vi "Handle Remote Command.vi"(8 "error in (no error)":errorcluster, 9 "Data":string, 10 "Command":string, 11 "Instrument in":refnum<class "Instrument.lvclass">) -> (0 "error out":errorcluster, 2 "String":string, 3 "Instrument out":refnum<class "Instrument.lvclass">)   [LabVIEW 2016, in "Instrument.lvclass"]
uses:
  Instrument.lvclass
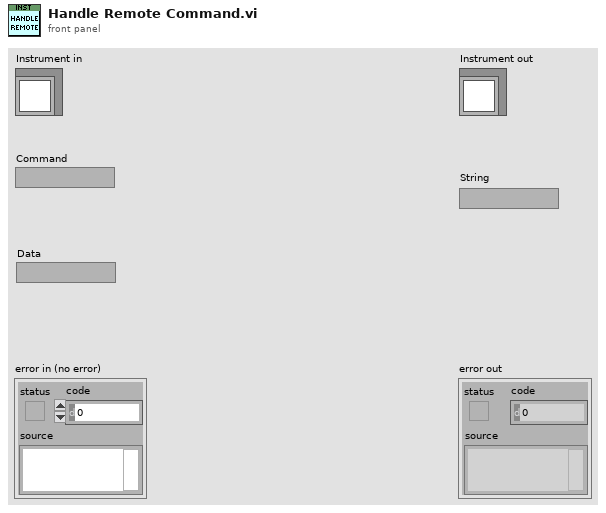
[diagram p1: front panel]
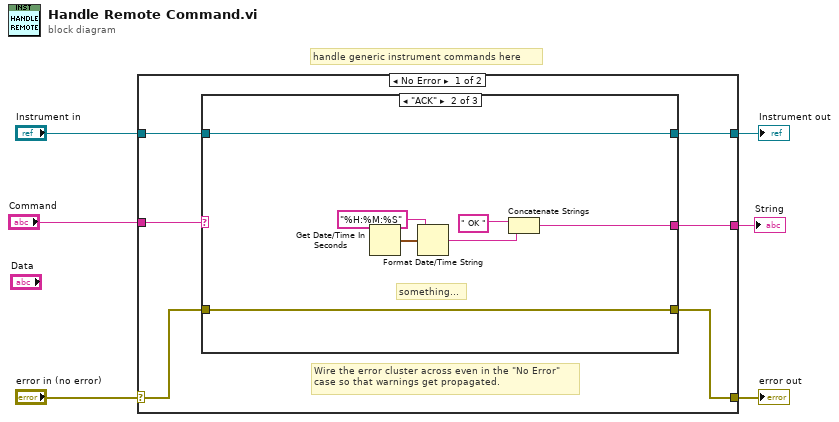
[diagram p0: block diagram]
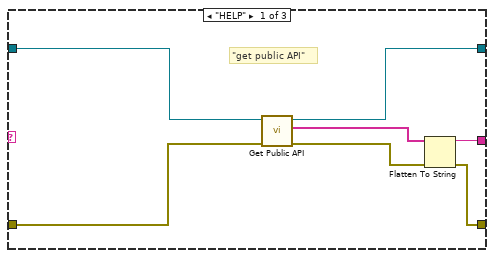
[diagram p2: hidden frame]
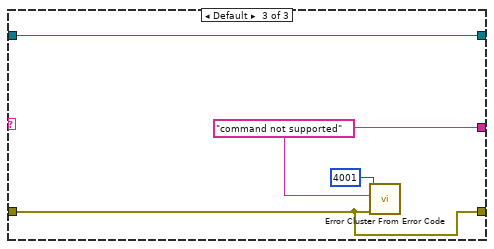
[diagram p3: hidden frame]
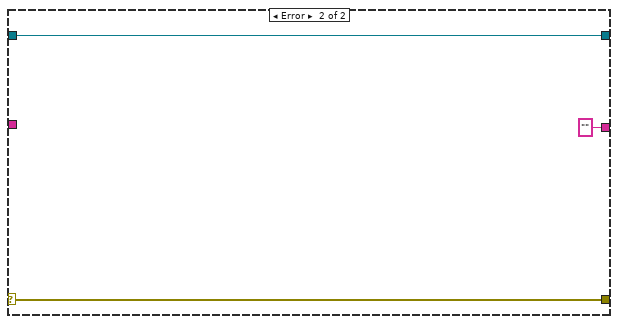
[diagram p4: hidden frame]
diagram:
  # "handle generic instrument commands here"
  n1 = case shown="No Error" "error in (no error)" {
    selector: "error in (no error)" -> [w8 w33]
    tunnel: [w7 w33] -> w5
    tunnel: [w10 w32] -> w3
    tunnel: "Instrument in" -> [w11 w32]
    tunnel: "Command" -> [w12 _]
    tunnel: [w9 "" ("error message (\"\")")] -> w1
    frame No Error {
      # "Wire the error cluster across even in the \"No Error\"\ncase so that warnings get propagated."
      n2 = case shown="\"ACK\"" w12 {
        tunnel: w11 -> [w19 w26 w29]
        tunnel: [w18 w26 w29] -> w10
        tunnel: [w15 w20 w27] -> w9
        tunnel: w8 -> [w17 w21 w28]
        tunnel: [w13 w21 w28] -> w7
        frame "HELP" {
          # "\"get public API\""
          n3 = call-dynamic "Get Public API.vi"("error in (no error)"=w17, "Instrument in"=w19) -> ("error out"=w14:errorcluster, "Commands"=w16:string[], "Instrument out"=w18:refnum<class "Instrument.lvclass">)  [unwired: 7 in]
          n4 = Flatten To String(anything=w16, error in (no error)=w14) -> (data string=w15:string, error out=w13:errorcluster)  [unwired: 2 in, 1 out]
        }
        frame "ACK" {
          # "something..."
          n5 = Get Date/Time In Seconds() -> (seconds since 1Jan1904=w23:timestamp)
          n6 = Format Date/Time String(time format string (%c)="%H:%M:%S", seconds (now)=w23) -> (date/time string=w24:string)  [unwired: 1 in]
          n7 = Concatenate Strings(" OK " ("data"), w24) -> (w20:string)
        }
        frame Default {
          w27 = "command not supported" ("error message (\"\")")
          n8 = call <vilib>:"Error Cluster From Error Code.vi"("error in (no error)"=w28, "error message (\"\")"=w27, "error code (0)"=4001) -> ()  [unwired: 6 in, 1 out]
        }
      }
    }
    frame Error {
    }
  }
  "error out" <- w5
  "Instrument out" <- w3
  "String" <- w1
